vi "Query Source Compliance Status.vi"(8 "error in (no error)":errorcluster, 10 "Source Measure Unit Channel (0: Channel A)":i32(ring) items=["Channel A", "Channel B"], 11 "VISA resource name":refnum<visa-resource-name>) -> (0 "error out":errorcluster, 2 "Compliance State":bool, 3 "VISA resource name out":refnum<visa-resource-name>)   [LabVIEW 2020, in "Keithley 2600 Series.lvlib"]
doc: "Returns the state of source compliance."
uses:
  <instrlib>/Keithley 2600 Series/Keithley 2600 Series.lvlib
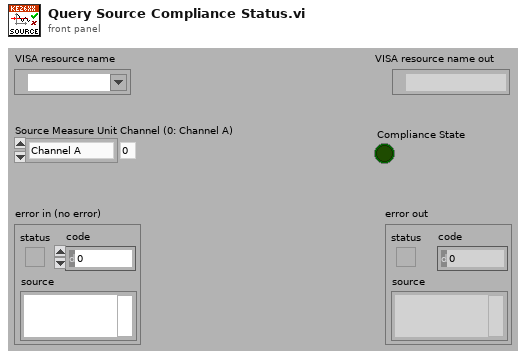
[diagram p1: front panel]
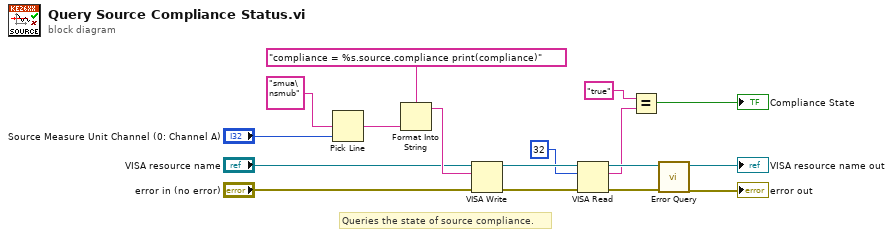
[diagram p0: block diagram]
diagram:
  # "Queries the state of source compliance."
  n1 = Pick Line(multi-line string="smua\nsmub", line index="Source Measure Unit Channel (0: Channel A)") -> (output string=w4:string)  [unwired: 1 in]
  n2 = Format Into String(format string="compliance = %s.source.compliance print(compliance)", w4) -> (resulting string=w16:string)  [unwired: 2 in, 1 out]
  n3 = VISA Write(VISA resource name="VISA resource name", write buffer=w16, error in (no error)="error in (no error)") -> (VISA resource name out=w11:refnum<visa-resource-name>, error out=w9:errorcluster)  [unwired: 1 out]
  n4 = VISA Read(VISA resource name=w11, byte count=u32 32, error in (no error)=w9) -> (VISA resource name out=w10:refnum<visa-resource-name>, read buffer=w3:string, error out=w8:errorcluster)  [unwired: 1 out]
  n5 = Equal?(x="true", y=w3) -> (x = y?=→"Compliance State":bool)
  n6 = call <instrlib>:"Error Query.vi"("error in (no error)"=w8, "VISA resource name"=w10) -> ("error out"=→"error out":errorcluster, "VISA resource name out"=→"VISA resource name out":refnum<visa-resource-name>)  [unwired: 6 in, 2 out]
